vi "FreqResponseLab10.vi"() -> ()   [LabVIEW 2021]
uses:
  <vilib>/Instr/_visa.llb/VISA Flush IO Buffer Mask.ctl
  <vilib>/Instr/_visa.llb/VISA Configure Serial Port (Instr).vi
  <vilib>/Utility/file.llb/Write Delimited Spreadsheet (DBL).vi
panel:
  out "error out 3":errorcluster
  in  "START":bool
  out "output array":dbl[][](array[numeric])
  in  "No.Plotpoints":i32
  in  "Min Frequency":dbl
  in  "Max Frequency":dbl
  out "current iteration":dbl[](array[numeric])
  # "Remember to change your com port to match the port used by your IBM4"
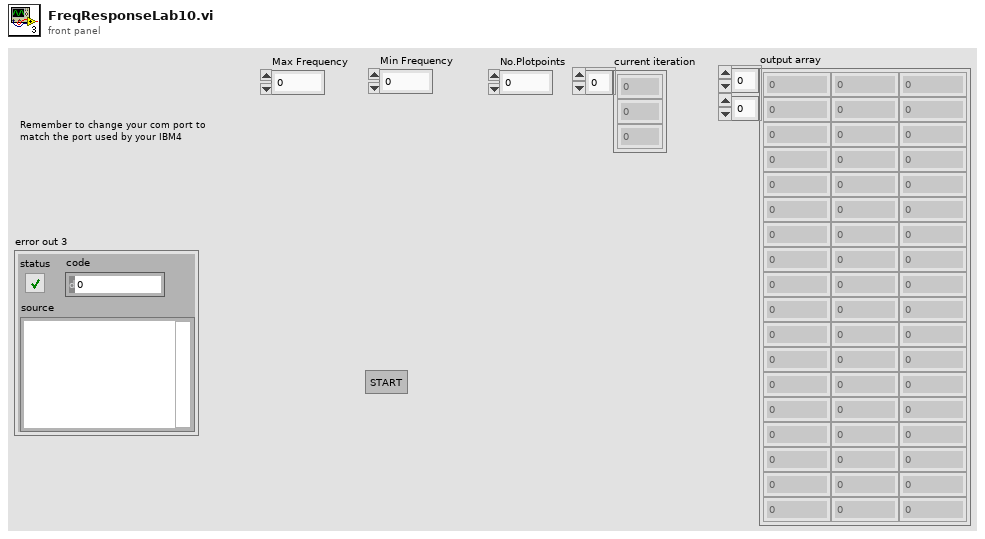
[diagram p1: front panel]
types:
  T1 = typedef "VISA Flush IO Buffer Mask.ctl" = u16
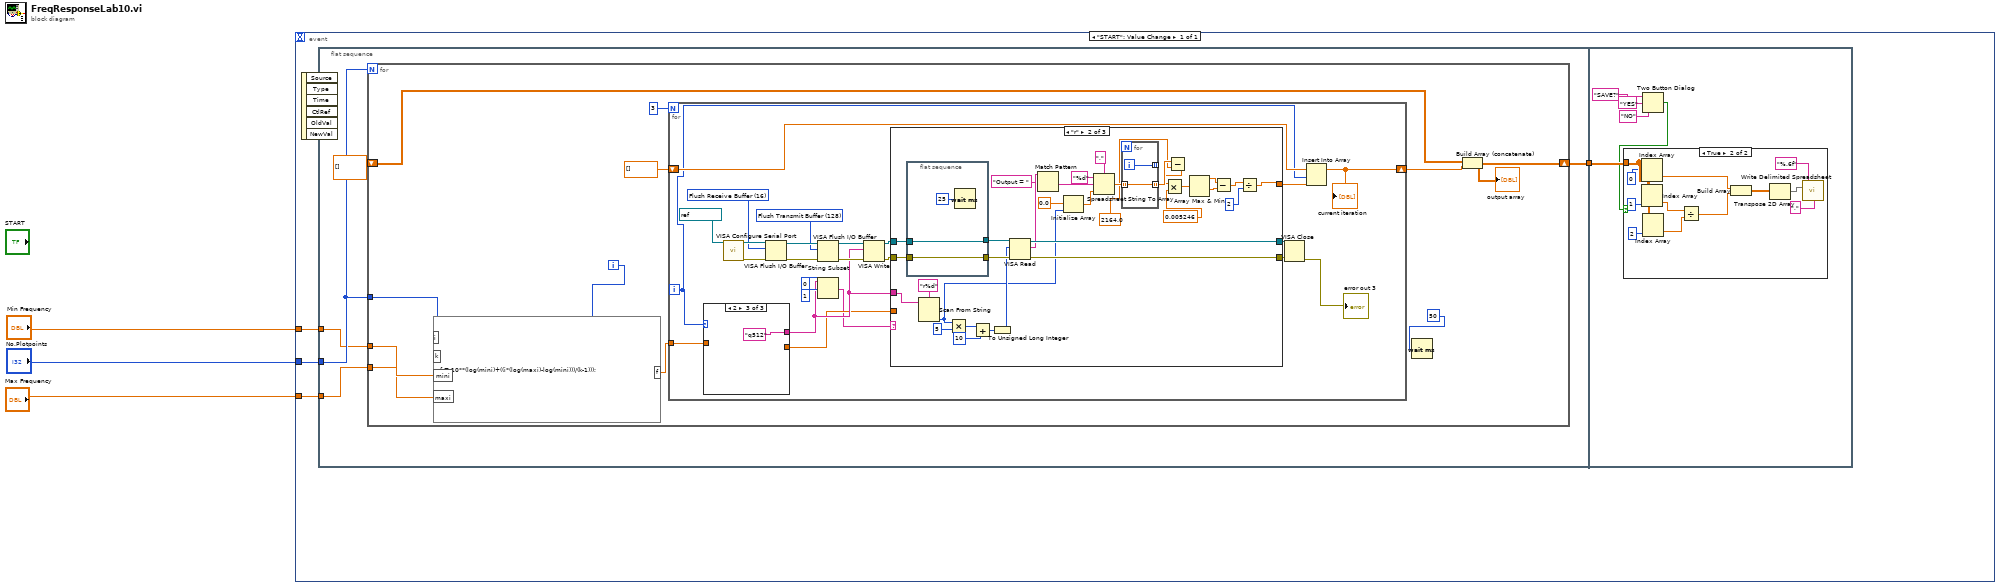
[diagram p0: block diagram]
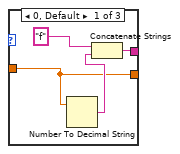
[diagram p2: hidden frame]
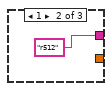
[diagram p3: hidden frame]
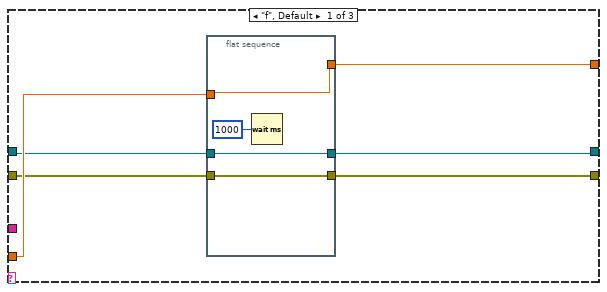
[diagram p4: hidden frame]
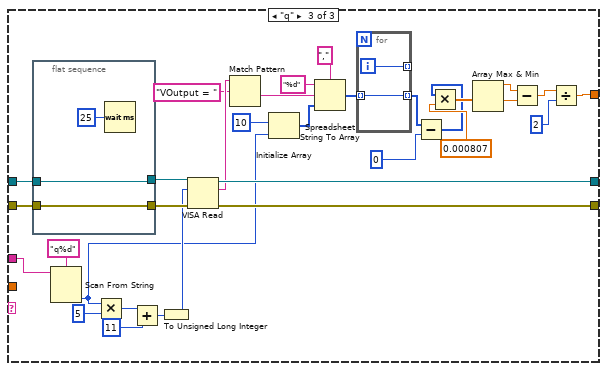
[diagram p5: hidden frame]
diagram:
  n1 = event shown="[0] \"START\": Value Change" {
    selector: _ -> [_]
    dyn-events: _ -> [_]
    timeout: _ -> [_]
    tunnel: "No.Plotpoints" -> [w7]
    tunnel: "Min Frequency" -> [w6]
    tunnel: "Max Frequency" -> [w5]
    event "START": Value Change {
      n2 = event-data() -> ()  [unwired: 1 in, 6 out]
      n3 = flat-sequence {
        tunnel: w7 -> [w12]
        tunnel: w6 -> [w11]
        tunnel: w5 -> [w10]
        tunnel: [w8] -> w4
        tunnel: w4 -> [w142]
        frame #0 {
          n4 = for {
            N: w12 -> [_]
            tunnel: w12 -> [w19]
            tunnel: w11 -> [w18]
            tunnel: w10 -> [w17]
            shift-right: [w14] -> w8
            shift-left: dbl[][] [] -> [w13]
            i -> [w20]
            n5 = formula code="f = 10**(log(mini)+((i*(log(maxi)-log(mini)))/(k-1)));"("i"=w20, "k"=w19, "mini"=w18, "maxi"=w17) -> ("f"=w16:dbl)
            n6 = for {
              N: 3 -> [_]
              shift-right: [w25] -> w15
              shift-left: dbl[] [] -> [w29]
              tunnel: w16 -> [w26]
              i -> [w28]
              w41 = T1 128 items=["Flush Receive Buffer"=16, "Write Transmit Buffer to Device"=32, "Flush Receive Buffer (No I/O)"=64, "Flush Transmit Buffer"=128] ("Mask")
              w44 = T1 16 items=["Flush Receive Buffer"=16, "Write Transmit Buffer to Device"=32, "Flush Receive Buffer (No I/O)"=64, "Flush Transmit Buffer"=128] ("Mask")
              n7 = case shown="2" w28 {
                tunnel: [w50 "r512" "q512"] -> w33
                tunnel: [w48 _ _] -> w32
                tunnel: w26 -> [w48 _ _]
                frame 0, Default {
                  n8 = Number To Decimal String(number=w48) -> (decimal integer string=w49:string)  [unwired: 1 in]
                  n9 = Concatenate Strings("f", w49) -> (w50:string)
                }
                frame 1 {
                }
                frame 2 {
                }
              }
              n10 = call-poly "VISA Configure Serial Port"("VISA resource name"=refnum<visa-resource-name> "COM5") -> ("VISA resource name out"=w46:refnum<visa-resource-name>, "error out"=w45:errorcluster)  [unwired: 13 in]
              n11 = VISA Flush I/O Buffer(VISA resource name=w46, mask (16)=w44, error in (no error)=w45) -> (VISA resource name out=w43:refnum<visa-resource-name>, error out=w42:errorcluster)
              n12 = VISA Flush I/O Buffer(VISA resource name=w43, mask (16)=w41, error in (no error)=w42) -> (VISA resource name out=w40:refnum<visa-resource-name>, error out=w39:errorcluster)
              n13 = String Subset(string=w33, offset (0)=0, length (rest)=1 ("length (rest)")) -> (substring=w31:string)
              n14 = VISA Write(VISA resource name=w40, write buffer=w33, error in (no error)=w39) -> (VISA resource name out=w37:refnum<visa-resource-name>, error out=w36:errorcluster)  [unwired: 1 out]
              n15 = case shown="\"r\"" w31 {
                tunnel: [w54 w95 w132] -> w38
                tunnel: [w56 w94 w131] -> w27
                tunnel: w37 -> [w57 w93 w130]
                tunnel: w36 -> [w55 w91 w128]
                tunnel: w33 -> [_ w89 w126]
                tunnel: w32 -> [w59 _ _]
                tunnel: [w58 w70 w106] -> w30
                frame "f", Default {
                  n16 = flat-sequence {
                    tunnel: w59 -> [w62]
                    tunnel: [w62] -> w58
                    tunnel: [w61] -> w56
                    tunnel: w57 -> [w61]
                    tunnel: w55 -> [w60]
                    tunnel: [w60] -> w54
                    frame #0 {
                      n17 = Wait (ms)(milliseconds to wait=u32 1000) -> ()  [unwired: 1 out]
                    }
                  }
                }
                frame "r" {
                  n18 = flat-sequence {
                    tunnel: [w100] -> w92
                    tunnel: w93 -> [w100]
                    tunnel: [w99] -> w90
                    tunnel: w91 -> [w99]
                    frame #0 {
                      n19 = Wait (ms)(milliseconds to wait=u32 25) -> ()  [unwired: 1 out]
                    }
                  }
                  n20 = Scan From String(format string="r%d", input string=w89) -> (output 1=w77:i32)  [unwired: 3 in, 3 out]
                  n21 = Multiply(x=w77, y=5) -> (x*y=w86:i32)
                  n22 = Add(x=w86, y=10) -> (x+y=w84:i32)
                  n23 = To Unsigned Long Integer(number=w84) -> (unsigned 32bit integer=w83:u32)
                  n24 = VISA Read(VISA resource name=w92, byte count=w83, error in (no error)=w90) -> (VISA resource name out=w94:refnum<visa-resource-name>, read buffer=w82:string, error out=w95:errorcluster)  [unwired: 1 out]
                  n25 = Match Pattern(string=w82, regular expression="Output = ") -> (after substring=w80:string)  [unwired: 1 in, 3 out]
                  n26 = Initialize Array(0.0, w77) -> (w76:dbl[])
                  n27 = Spreadsheet String To Array(delimiter (Tab)=",", format string="%d", spreadsheet string=w80, array type (2D Dbl)=w76) -> (array=w75:dbl[])
                  n28 = for {
                    tunnel: w75 -> [w97] mode=indexing
                    tunnel: [w97] -> w66 mode=indexing
                    tunnel: [w96] -> _ mode=indexing
                    i -> [w96]
                  }
                  n29 = Subtract(x=w66, y=2164.0) -> (x-y=w64:dbl[])
                  n30 = Multiply(x=w64, y=0.005246) -> (x*y=w69:dbl[])
                  n31 = Array Max & Min(array=w69) -> (max value=w74:dbl, min value=w73:dbl)  [unwired: 2 out]
                  n32 = Subtract(x=w74, y=w73) -> (x-y=w72:dbl)
                  n33 = Divide(x=w72, y=2) -> (x/y=w70:dbl)
                }
                frame "q" {
                  n34 = flat-sequence {
                    tunnel: [w137] -> w129
                    tunnel: w130 -> [w137]
                    tunnel: [w136] -> w127
                    tunnel: w128 -> [w136]
                    frame #0 {
                      n35 = Wait (ms)(milliseconds to wait=u32 25) -> ()  [unwired: 1 out]
                    }
                  }
                  n36 = Scan From String(format string="q%d", input string=w126) -> (output 1=w113:i32)  [unwired: 3 in, 3 out]
                  n37 = Multiply(x=w113, y=5) -> (x*y=w123:i32)
                  n38 = Add(x=w123, y=11) -> (x+y=w121:i32)
                  n39 = To Unsigned Long Integer(number=w121) -> (unsigned 32bit integer=w120:u32)
                  n40 = VISA Read(VISA resource name=w129, byte count=w120, error in (no error)=w127) -> (VISA resource name out=w131:refnum<visa-resource-name>, read buffer=w119:string, error out=w132:errorcluster)  [unwired: 1 out]
                  n41 = Match Pattern(string=w119, regular expression="VOutput = ") -> (after substring=w117:string)  [unwired: 1 in, 3 out]
                  n42 = Initialize Array(10 ("y"), w113) -> (w112:i32[])
                  n43 = Spreadsheet String To Array(delimiter (Tab)=",", format string="%d", spreadsheet string=w117, array type (2D Dbl)=w112) -> (array=w111:i32[])
                  n44 = for {
                    tunnel: w111 -> [w134] mode=indexing
                    tunnel: [w134] -> w103 mode=indexing
                    tunnel: [w133] -> _ mode=indexing
                    i -> [w133]
                  }
                  n45 = Subtract(x=w103, y=0) -> (x-y=w101:i32[])
                  n46 = Multiply(x=w101, y=0.000807) -> (x*y=w105:dbl[])
                  n47 = Array Max & Min(array=w105) -> (max value=w110:dbl, min value=w109:dbl)  [unwired: 2 out]
                  n48 = Subtract(x=w110, y=w109) -> (x-y=w108:dbl)
                  n49 = Divide(x=w108, y=2) -> (x/y=w106:dbl)
                }
              }
              n50 = VISA Close(VISA resource name=w27, error in (no error)=w38) -> (error out=→"error out 3":errorcluster)
              n51 = Insert Into Array(array=w29, index=w28, new element=w30) -> (w25:dbl[])
              "current iteration" <- w25
            }
            n52 = Wait (ms)(milliseconds to wait=u32 50) -> ()  [unwired: 1 out]
            n53 = Build Array (concatenate)(w13, w15) -> (w14:dbl[][])
            "output array" <- w14
          }
        }
        frame #1 {
          n54 = Two Button Dialog(message="SAVE?", 1:"NO" ("F button name (\"Cancel\")"), 2:"YES" ("T button name (\"OK\")")) -> (T button?=w138:bool)
          n55 = case shown="True" w138 {
            tunnel: w142 -> [_ w146]
            frame False {
            }
            frame True {
              n56 = Index Array(array=w146, index (col)=0 ("disabled index (col)")) -> (element=w150:dbl[])  [unwired: 1 in]
              n57 = Index Array(array=w146, index (col)=1 ("disabled index (col)")) -> (element=w149:dbl[])  [unwired: 1 in]
              n58 = Index Array(array=w146, index (col)=2 ("disabled index (col)")) -> (element=w154:dbl[])  [unwired: 1 in]
              n59 = Divide(x=w149, y=w154) -> (x/y=w151:dbl[])
              n60 = Build Array(w150, w151) -> (w152:dbl[][])
              n61 = Transpose 2D Array(2D array=w152) -> (transposed array=w153:dbl[][])
              n62 = call-poly <vilib>:"Write Delimited Spreadsheet.vi"("format (%.3f)"="%.6f", "2D data"=w153, "delimiter (\\t)"="," ("delimiter (\\t)")) -> ()  [unwired: 11 in, 2 out]
            }
          }
        }
      }
    }
  }
